vi "getEventSummaryState.vi"(8 "error in (no error)":errorcluster, 11 "SALCommunicatorView in":refnum<class "SALCommunicatorView.lvclass">) -> (0 "error out":errorcluster, 1 "SummaryStateValue":i32, 2 "function return":i32, 3 "SALCommunicatorView out":refnum<class "SALCommunicatorView.lvclass">)   [LabVIEW 2016, in "SALCommunicatorTC.lvclass"]
uses:
  SALCommunicatorTC/SALCommunicatorTC.lvclass
  SALCommunicatorView.lvclass
  ts_sallv_exa/SALLV_EXA.lvlib
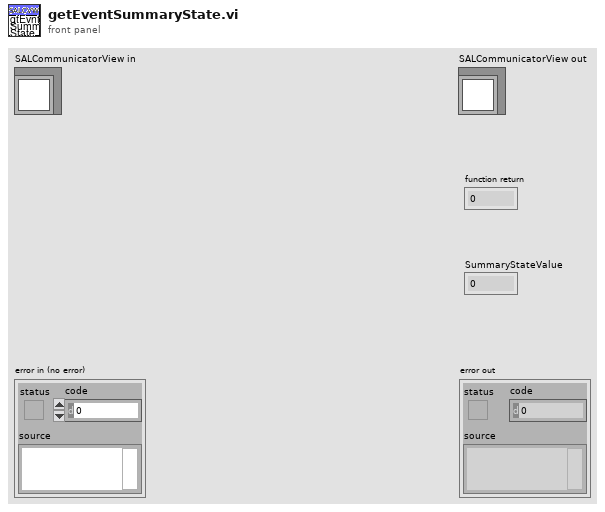
[diagram p1: front panel]
types:
  T1 = typedef "SALLV_EXA.lvlib/logevent_SummaryState.ctl" = cluster{"SummaryStateValue":i32, "priority":i32}
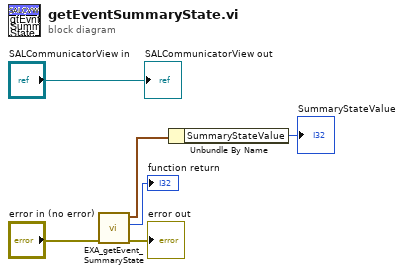
[diagram p0: block diagram]
diagram:
  n1 = call "EXA_getEvent_SummaryState.vi"("error in (no error)"="error in (no error)") -> ("error out"=→"error out":errorcluster, "function return"=→"function return":i32, "logevent_SummaryState_Ctl out"=w2:T1)  [unwired: 8 in]
  n2 = Unbundle By Name(w2) -> ("SummaryStateValue"=→"SummaryStateValue":i32)
  "SALCommunicatorView out" <- "SALCommunicatorView in"
